vi "Manual_TEST_KBS.vi"() -> ()   [LabVIEW 2018]
uses:
  <vilib>/Instr/_visa.llb/VISA Configure Serial Port (Instr).vi
panel:
  out "read buffer":string
  in  "Comport":refnum<visa-resource-name>
  in  "Brake":u8
  in  "E-Stop":bool
  in  "M/A":bool
  in  "Steering(deg)":i16(knob) scale=-2000.0..2000.0
  in  "Speed":u16
  in  "F_B":u8
  in  "stop":bool
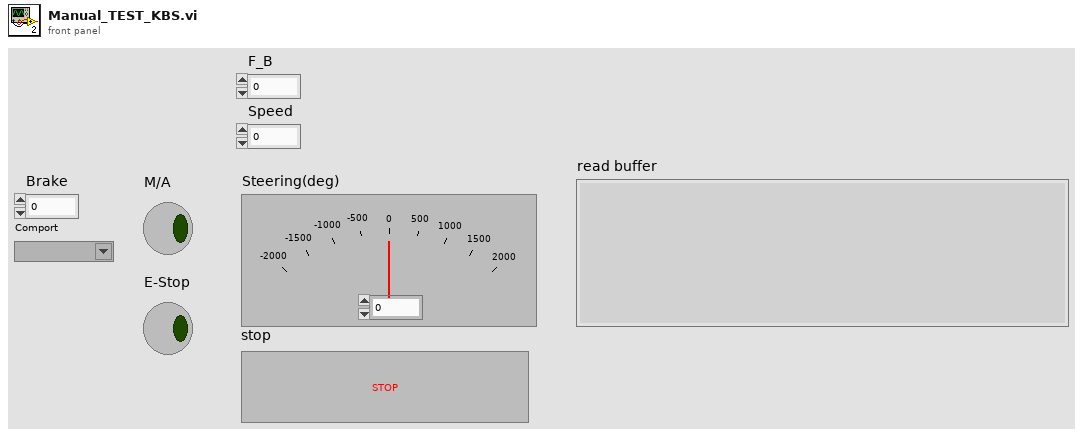
[diagram p1: front panel]
types:
  T1 = cluster{"AorM":u8, "E-Stop":u8, "F_B":u8, "Speed":u16, "Steer":i16, "Brake":u8, "Encoder":u8, "Encoder 2":u8, "Encoder 3":u8, "Encoder 4":u8, "ALIVE":u8, "ETX_0":u8, "ETX_0 2":u8}
  T2 = cluster{"S":u8, "T":u8, "X":u8, "AorM":u8, "E-Stop":u8, "F_B":u8, "Speed":u16, "Steer":i16, "Brake":u8, "ALIVE":u8, "ETX_0":u8, "ETX_0 2":u8}
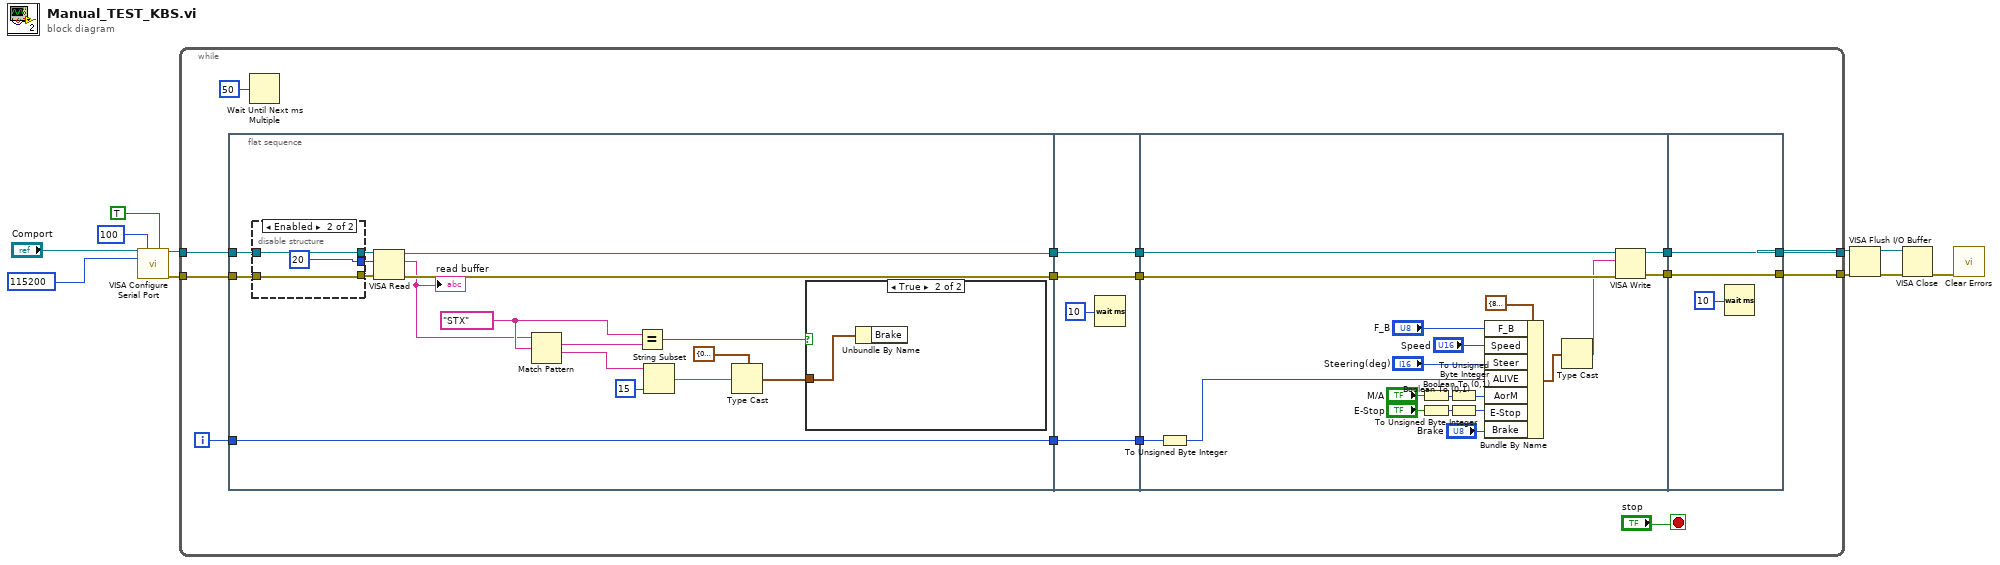
[diagram p0: block diagram]
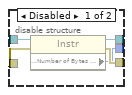
[diagram p2: hidden frame]
diagram:
  n1 = call-poly "VISA Configure Serial Port"("VISA resource name"="Comport", "timeout (10sec)"=u32 100, "Enable Termination\nChar (T)"=TRUE ("Enable Termination\nChar (T)"), "baud rate (9600)"=u32 115200) -> ("VISA resource name out"=w4:refnum<visa-resource-name>, "error out"=w3:errorcluster)  [unwired: 10 in]
  n2 = while {
    tunnel: w4 -> [w25]
    tunnel: w3 -> [w24]
    tunnel: [w22] -> w6
    tunnel: [w21] -> w5
    i -> [w23]
    stop <- "stop" stop-if-true
    n3 = flat-sequence {
      tunnel: w25 -> [w43]
      tunnel: w24 -> [w42]
      tunnel: [w41] -> w20
      tunnel: [w40] -> w18
      tunnel: w23 -> [w39]
      tunnel: [w39] -> w16
      tunnel: w20 -> [w56]
      tunnel: [w56] -> w19
      tunnel: w18 -> [w55]
      tunnel: [w55] -> w17
      tunnel: w16 -> [w54]
      tunnel: [w54] -> w15
      tunnel: w19 -> [w73]
      tunnel: w17 -> [w72]
      tunnel: w15 -> [w70]
      tunnel: [w69] -> w14
      tunnel: [w68] -> w13
      tunnel: [w77] -> w21
      tunnel: [w78] -> w22
      tunnel: w14 -> [w78]
      tunnel: w13 -> [w77]
      frame #0 {
        w33 = "STX" ("검색 문자열/문자 (-)")
        n4 = disable-structure shown="Enabled" {
          disable-tunnel: w43 -> [w48 w50]
          disable-tunnel: w42 -> [w47 w51]
          disable-tunnel: [w46 w51] -> w38
          disable-tunnel: [w45 u32 20 ("timeout (10sec)")] -> w37
          disable-tunnel: [w44 w50] -> w36
          frame Disabled {
            n5 = property class="Instr"(reference=w48, error in=w47) -> (reference out=w44:refnum<visa-resource-name>, error out=w46:errorcluster, "Serial Settings:Number of Bytes at Serial Port"=w45:u32)
          }
          frame Enabled {
          }
        }
        n6 = VISA Read(VISA resource name=w36, byte count=w37, error in (no error)=w38) -> (VISA resource name out=w41:refnum<visa-resource-name>, read buffer=w31:string, error out=w40:errorcluster)  [unwired: 1 out]
        "read buffer" <- w31
        n7 = Match Pattern(string=w31, regular expression=w33) -> (match substring=w32:string, after substring=w35:string)  [unwired: 1 in, 2 out]
        n8 = Equal?(x=w33, y=w32) -> (x = y?=w30:bool)
        n9 = String Subset(string=w35, length (rest)=15 ("길이(나머지)")) -> (substring=w29:string)  [unwired: 1 in]
        n10 = Type Cast(type=T1 {"AorM"=0, "E-Stop"=0, "F_B"=0, "Speed"=0, "Steer"=0, "Brake"=0, "Encoder"=0, "Encoder 2"=0, "Encoder 3"=0, "Encoder 4"=0, "ALIVE"=0, "ETX_0"=13, "ETX_0 2"=10}, x=w29) -> (*(type *) &x=w28:T1)
        n11 = case shown="True" w30 {
          tunnel: w28 -> [_ w52]
          frame False {
          }
          frame True {
            n12 = Unbundle By Name(w52) -> ()  [unwired: 1 out]
          }
        }
      }
      frame #1 {
        n13 = Wait (ms)(milliseconds to wait=u32 10 ("대기 시간(ms)")) -> ()  [unwired: 1 out]
      }
      frame #2 {
        n14 = To Unsigned Byte Integer(number=w70) -> (unsigned 8bit integer=w75:u8)
        n15 = Boolean To (0,1)(Boolean="M/A") -> (0, 1=w62:i16)
        n16 = Boolean To (0,1)(Boolean="E-Stop") -> (0, 1=w60:i16)
        n17 = To Unsigned Byte Integer(number=w62) -> (unsigned 8bit integer=w61:u8)
        n18 = To Unsigned Byte Integer(number=w60) -> (unsigned 8bit integer=w58:u8)
        n19 = Bundle By Name(cluster=T2 {"S"=83, "T"=84, "X"=88, "AorM"=0, "E-Stop"=0, "F_B"=0, "Speed"=0, "Steer"=0, "Brake"=0, "ALIVE"=0, "ETX_0"=13, "ETX_0 2"=10}, "F_B"="F_B", "Speed"="Speed", "Steer"="Steering(deg)", "ALIVE"=w75, "AorM"=w61, "E-Stop"=w58, "Brake"="Brake") -> (w74:T2)
        n20 = Type Cast(x=w74) -> (*(type *) &x=w71:string)  [unwired: 1 in]
        n21 = VISA Write(VISA resource name=w73, write buffer=w71, error in (no error)=w72) -> (VISA resource name out=w69:refnum<visa-resource-name>, error out=w68:errorcluster)  [unwired: 1 out]
      }
      frame #3 {
        n22 = Wait (ms)(milliseconds to wait=u32 10 ("대기 시간(ms)")) -> ()  [unwired: 1 out]
      }
    }
    n23 = Wait Until Next ms Multiple(millisecond multiple=u32 50 ("ms 배수")) -> ()  [unwired: 1 out]
  }
  n24 = VISA Flush I/O Buffer(VISA resource name=w6, error in (no error)=w5) -> (VISA resource name out=w7:refnum<visa-resource-name>, error out=w8:errorcluster)  [unwired: 1 in]
  n25 = VISA Close(VISA resource name=w7, error in (no error)=w8) -> (error out=w2:errorcluster)
  n26 = call <vilib>:"Clear Errors.vi"("error in (no error)"=w2) -> ()  [unwired: 5 in, 2 out]
